vi "Get Status.vi"(8 "error in (no error)":errorcluster, 10 "Header Contents in":T1={"FILENAME"=["FILENAME", "example.fits", "File name at acquisition"], "OBSERVER"=["OBSERVER", "ECHARPE", "PI name"], "PROGRID"=["PROGRID", "UNDEFINED", "Program ID"], "OBJECT"=["OBJECT", "UNDEFINED", "Object name"], "NIGHTDIR"=["NIGHTDIR", "C:\\Users\\Sparc4_2\\Desktop\\Software Echarpe\\Imagens", "Night directory name "], "CHANNEL"=["CHANNEL", "RED", "Instrument channel"], "INSTRUME"=["INSTRUME", "ECHARPE", "Instrument"], "NEXPSEQ"=["NEXPSEQ", "1", "Total number of exposures in sequence"], "SEQINDEX"=["SEQINDEX", "1", "Exposure index in the sequence"], "OBSTYPE"=["OBSTYPE", "BIAS", "Image type: OBJECT, BIAS, FLAT, ARC, DARK"], "READMOD"=["READMOD", "Normal", "Read out mode: fast, normal, slow"], "SHUTTER"=["SHUTTER", "CLOSED", "Shutter Mode (OPEN, CLOSED, or AUTO) "], "OPENSHT"=["OPENSHT", "50", "Time to open the shutter (ms) "], "CLOSESHT"=["CLOSESHT", "50", "Time to close the shutter (ms)"], "GAIN"=["GAIN", "3.38", "Gain (e-/ADU)"], "GAINERR "=["GAINERR", "0.05", " Gain error (e-/ADU)"], "RDNOISE"=["RDNOISE", "6.55", "Read noise (e-)"], "RNOISERR"=["RNOISERR", "0.02", "Read noise error (e-)"], "SKYFIBER"=["SKYFIBER", "OFF", "Sky fiber: ON or OFF"], "CALFIBER"=["CALFIBER", "OFF", "Calibration Fiber: ON or OFF"], "UTDATE"=["UTDATE", "2017-10-01T20", "UT date at start of exposure"], "LOCTIME"=["LOCTIME", "2017-10-01T17", "LT date at start of exposure"], "MJD"=["MJD", "58027.500000", "Modified Julian Date at start of exposure"], "OBSLON"=["OBSLON", "-45.57972", "Observatory East Longitude"], "OBSLAT"=["OBSLAT", "-22.53444", "Observatory Latitude"], "OBSALT"=["OBSALT", "1864.0", "Observatory elevation above sea level (m)"], "EXPTIME"=["EXPTIME", "1", "Exposure time (s)"], "TELRA"=["TELRA", "", "TCS right ascension: HH:MM:SS.SSS"], "TELDEC"=["TELDEC", "", "TCS declination: “+-DD:MM:SS.SSS”"], "RA"=["RA", "00:00:00.000", "Requested right Ascension: HH:MM:SS.SSS"], "DEC"=["DEC", "+00:00:00.000", "Requested Declination: +- DD:MM:SS.SSS"], "RA_DEG"=["RA_DEG", "", "Requested Right Ascension (deg)"], "DEC_DEG"=["DEC_DEG", "", "Requested Declination (deg)"], "EPOCH"=["EPOCH", "", "Epoch for Target coordinates"], "HA"=["HA", "+01:13:05.98", "Hour Angle (Sexagesimal)"], "HAD"=["HAD", "", "Hour Angle (deg)"], "AIRMASS"=["AIRMASS", "1.085", "Mean airmass for the observation"], "AMSTART"=["AMSTART", "", "Airmass at start of exposure"], "AMEND"=["AMEND", "", "Airmass at end of exposure"], "XOFFSET"=["XOFFSET", "", "Telescope RA offset in arcsec"], "YOFFSET"=["YOFFSET", "", "Telescope DEC offset in arcsec"], "PA"=["PA", "14.6415392418", "Current Rotator Position Angle (degree)"], "CAMFOC"=["CAMFOC", "-3.53", "Camera focus position (mm)"], "TELFOC"=["TELFOC", "-3.53", "Telescope focus position (mm)"], "TCSUT"=["TCSUT", "", "TCS Universal Time"], "MOONDIST"=["MOONDIST", "", "Moon angular distance to object (deg)"], "MOONALT"=["MOONALT", "", "Moon elevation above horizon (deg)"], "MONNPHAS"=["MOONPHAS", "2017-10-01T20:34:3 6.000", "Moon phase (deg)"], "ADC"=["ADC", "ON", "Atmospheric Dispersion Corrector: ON or OFF"], "ADCSPPED"=["ADCSPPED", "5.0", "ADC motor speed (rpm)"], "CALMIRR"=["CALMIRR", "OUT", "Calibration mirror position: IN or OUT"], "GUIDING"=["GUIDING", "ON", "Guider status: ON or OFF"], "GUIDTEXP"=["GUIDTEXP", "1.0", "Guider exposure time (s)"], "GUIDFREQ"=["GUIDFREQ", "1.0", "Guiding frequency (Hz)"], "GUIDOBJX"=["GUIDOBJX", "102.5", "Guiding object x position (pixel)"], "GUIDOBJY"=["GUIDOBJY", "300.3", "Guiding object y position (pixel)"], "AVGYCORR"=["AVGYCORR", "2.3", "Average correction in RA (arcsec)"], "AVGXCORR"=["AVGXCORR", "1.3", "Average correction in DEC (arcsec)"], "GFOCUS"=["GFOCUS", "3.0", "Guider focus position (mm)"], "THARLAMP"=["THARLAMP", "OFF", "Thorium-Argon lamp state: ON or OFF"], "HALLAMP"=["HALLAMP", "OFF", "Halogen lamp state: ON or OFF"], "AGITATOR"=["AGITATOR", "ON", "Fiber agitator: ON or OFF"], "THARMIRR"=["THARMIRR", "SPECTROGRAPH", "Th-Ar mirror position: SPECTROGRAPH or TELESCOPE"], "DSTATUS"=["DSTATUS", "OPEN", "Dome Status: OPEN or CLOSED"], "DTEMP"=["DTEMP", "10.0", "Dome temperature (deg C)"], "DHUM"=["DHUM", "82.0", "Dome humidity (per cent)"], "DLAMP"=["DLAMP", "OFF", "Dome lamp: ON or OFF"], "DFLAT"=["DFLAT", "OFF", "Dome flat lamp: ON or OFF"], "TEMPEXT"=["TEMPEXT", "10.0", "External temperature (deg C)"], "PRESSURE"=["PRESSURE", "742.00", "Pressure (mbar)"], "HUMIDITY"=["HUMIDITY", "92.00", "Humidity (per cent)"], "WINDDIR"=["WINDDIR", "15.0", "Wind direction: North-eastward (deg)"], "WSPEED"=["WSPEED", "30.2", "Wind Speed (km/h)"], "TCSST"=["TCSST", "2017-10-01T20:34:3 6.000", "TCS Sideral Time"], "DPOS"=["DPOS", "0.00000", "Dome position (deg)"]}, 11 "TCS in":refnum<class "TCS.lvclass">) -> (0 "error out":errorcluster, 2 "Header Contents out":T1={"FILENAME"=["FILENAME", "example.fits", "File name at acquisition"], "OBSERVER"=["OBSERVER", "ECHARPE", "PI name"], "PROGRID"=["PROGRID", "UNDEFINED", "Program ID"], "OBJECT"=["OBJECT", "UNDEFINED", "Object name"], "NIGHTDIR"=["NIGHTDIR", "C:\\Users\\Sparc4_2\\Desktop\\Software Echarpe\\Imagens", "Night directory name "], "CHANNEL"=["CHANNEL", "RED", "Instrument channel"], "INSTRUME"=["INSTRUME", "ECHARPE", "Instrument"], "NEXPSEQ"=["NEXPSEQ", "1", "Total number of exposures in sequence"], "SEQINDEX"=["SEQINDEX", "1", "Exposure index in the sequence"], "OBSTYPE"=["OBSTYPE", "BIAS", "Image type: OBJECT, BIAS, FLAT, ARC, DARK"], "READMOD"=["READMOD", "Normal", "Read out mode: fast, normal, slow"], "SHUTTER"=["SHUTTER", "CLOSED", "Shutter Mode (OPEN, CLOSED, or AUTO) "], "OPENSHT"=["OPENSHT", "50", "Time to open the shutter (ms) "], "CLOSESHT"=["CLOSESHT", "50", "Time to close the shutter (ms)"], "GAIN"=["GAIN", "3.38", "Gain (e-/ADU)"], "GAINERR "=["GAINERR", "0.05", " Gain error (e-/ADU)"], "RDNOISE"=["RDNOISE", "6.55", "Read noise (e-)"], "RNOISERR"=["RNOISERR", "0.02", "Read noise error (e-)"], "SKYFIBER"=["SKYFIBER", "OFF", "Sky fiber: ON or OFF"], "CALFIBER"=["CALFIBER", "OFF", "Calibration Fiber: ON or OFF"], "UTDATE"=["UTDATE", "2017-10-01T20", "UT date at start of exposure"], "LOCTIME"=["LOCTIME", "2017-10-01T17", "LT date at start of exposure"], "MJD"=["MJD", "58027.500000", "Modified Julian Date at start of exposure"], "OBSLON"=["OBSLON", "-45.57972", "Observatory East Longitude"], "OBSLAT"=["OBSLAT", "-22.53444", "Observatory Latitude"], "OBSALT"=["OBSALT", "1864.0", "Observatory elevation above sea level (m)"], "EXPTIME"=["EXPTIME", "1", "Exposure time (s)"], "TELRA"=["TELRA", "", "TCS right ascension: HH:MM:SS.SSS"], "TELDEC"=["TELDEC", "", "TCS declination: “+-DD:MM:SS.SSS”"], "RA"=["RA", "00:00:00.000", "Requested right Ascension: HH:MM:SS.SSS"], "DEC"=["DEC", "+00:00:00.000", "Requested Declination: +- DD:MM:SS.SSS"], "RA_DEG"=["RA_DEG", "", "Requested Right Ascension (deg)"], "DEC_DEG"=["DEC_DEG", "", "Requested Declination (deg)"], "EPOCH"=["EPOCH", "", "Epoch for Target coordinates"], "HA"=["HA", "+01:13:05.98", "Hour Angle (Sexagesimal)"], "HAD"=["HAD", "", "Hour Angle (deg)"], "AIRMASS"=["AIRMASS", "1.085", "Mean airmass for the observation"], "AMSTART"=["AMSTART", "", "Airmass at start of exposure"], "AMEND"=["AMEND", "", "Airmass at end of exposure"], "XOFFSET"=["XOFFSET", "", "Telescope RA offset in arcsec"], "YOFFSET"=["YOFFSET", "", "Telescope DEC offset in arcsec"], "PA"=["PA", "14.6415392418", "Current Rotator Position Angle (degree)"], "CAMFOC"=["CAMFOC", "-3.53", "Camera focus position (mm)"], "TELFOC"=["TELFOC", "-3.53", "Telescope focus position (mm)"], "TCSUT"=["TCSUT", "", "TCS Universal Time"], "MOONDIST"=["MOONDIST", "", "Moon angular distance to object (deg)"], "MOONALT"=["MOONALT", "", "Moon elevation above horizon (deg)"], "MONNPHAS"=["MOONPHAS", "2017-10-01T20:34:3 6.000", "Moon phase (deg)"], "ADC"=["ADC", "ON", "Atmospheric Dispersion Corrector: ON or OFF"], "ADCSPPED"=["ADCSPPED", "5.0", "ADC motor speed (rpm)"], "CALMIRR"=["CALMIRR", "OUT", "Calibration mirror position: IN or OUT"], "GUIDING"=["GUIDING", "ON", "Guider status: ON or OFF"], "GUIDTEXP"=["GUIDTEXP", "1.0", "Guider exposure time (s)"], "GUIDFREQ"=["GUIDFREQ", "1.0", "Guiding frequency (Hz)"], "GUIDOBJX"=["GUIDOBJX", "102.5", "Guiding object x position (pixel)"], "GUIDOBJY"=["GUIDOBJY", "300.3", "Guiding object y position (pixel)"], "AVGYCORR"=["AVGYCORR", "2.3", "Average correction in RA (arcsec)"], "AVGXCORR"=["AVGXCORR", "1.3", "Average correction in DEC (arcsec)"], "GFOCUS"=["GFOCUS", "3.0", "Guider focus position (mm)"], "THARLAMP"=["THARLAMP", "OFF", "Thorium-Argon lamp state: ON or OFF"], "HALLAMP"=["HALLAMP", "OFF", "Halogen lamp state: ON or OFF"], "AGITATOR"=["AGITATOR", "ON", "Fiber agitator: ON or OFF"], "THARMIRR"=["THARMIRR", "SPECTROGRAPH", "Th-Ar mirror position: SPECTROGRAPH or TELESCOPE"], "DSTATUS"=["DSTATUS", "OPEN", "Dome Status: OPEN or CLOSED"], "DTEMP"=["DTEMP", "10.0", "Dome temperature (deg C)"], "DHUM"=["DHUM", "82.0", "Dome humidity (per cent)"], "DLAMP"=["DLAMP", "OFF", "Dome lamp: ON or OFF"], "DFLAT"=["DFLAT", "OFF", "Dome flat lamp: ON or OFF"], "TEMPEXT"=["TEMPEXT", "10.0", "External temperature (deg C)"], "PRESSURE"=["PRESSURE", "742.00", "Pressure (mbar)"], "HUMIDITY"=["HUMIDITY", "92.00", "Humidity (per cent)"], "WINDDIR"=["WINDDIR", "15.0", "Wind direction: North-eastward (deg)"], "WSPEED"=["WSPEED", "30.2", "Wind Speed (km/h)"], "TCSST"=["TCSST", "2017-10-01T20:34:3 6.000", "TCS Sideral Time"], "DPOS"=["DPOS", "0.00000", "Dome position (deg)"]}, 3 "TCS out":refnum<class "TCS.lvclass">)   [LabVIEW 2018, in "TCS.lvclass"]
uses:
  TCS.lvclass
  TCS.lvclass/TCS.ctl
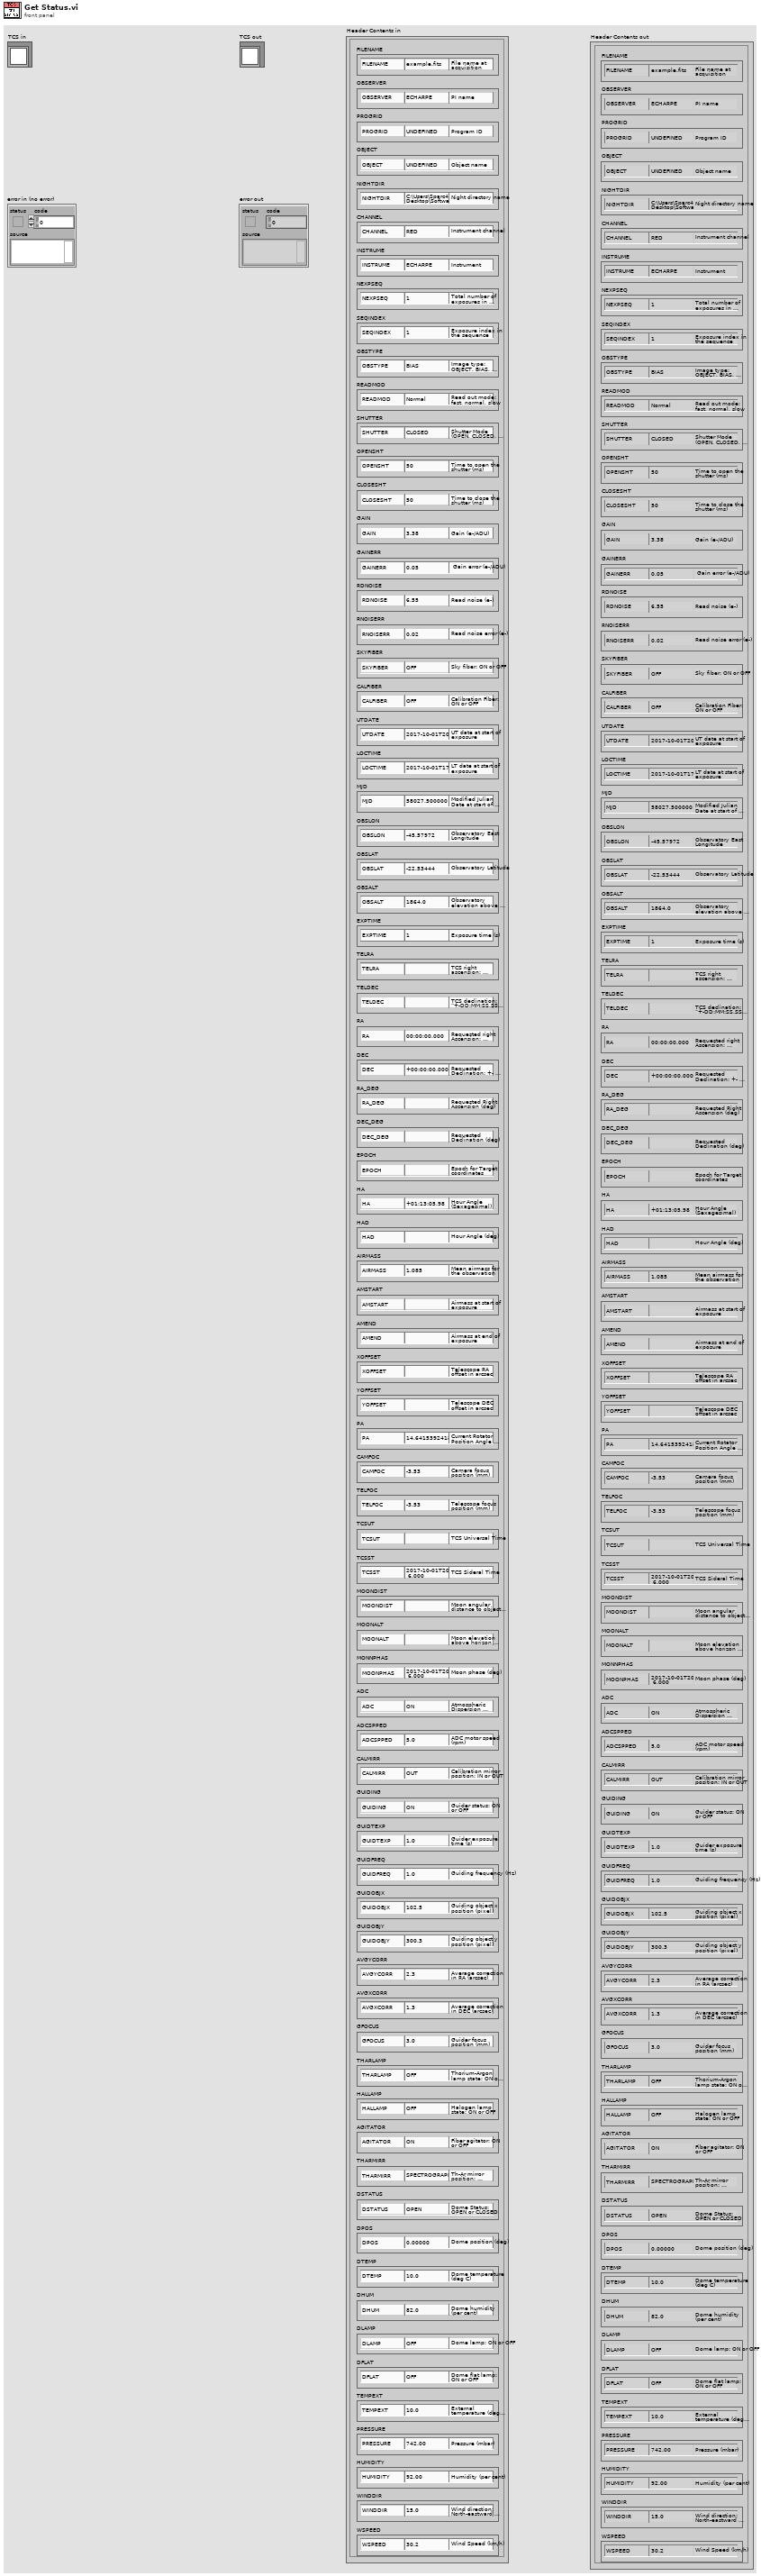
[diagram p1: front panel]
types:
  T1 = cluster{"FILENAME":string[], "OBSERVER":string[], "PROGRID":string[], "OBJECT":string[], "NIGHTDIR":string[], "CHANNEL":string[], "INSTRUME":string[], "NEXPSEQ":string[], "SEQINDEX":string[], "OBSTYPE":string[], "READMOD":string[], "SHUTTER":string[], "OPENSHT":string[], "CLOSESHT":string[], "GAIN":string[], "GAINERR ":string[], "RDNOISE":string[], "RNOISERR":string[], "SKYFIBER":string[], "CALFIBER":string[], "UTDATE":string[], "LOCTIME":string[], "MJD":string[], "OBSLON":string[], "OBSLAT":string[], "OBSALT":string[], "EXPTIME":string[], "TELRA":string[], "TELDEC":string[], "RA":string[], "DEC":string[], "RA_DEG":string[], "DEC_DEG":string[], "EPOCH":string[], "HA":string[], "HAD":string[], "AIRMASS":string[], "AMSTART":string[], "AMEND":string[], "XOFFSET":string[], "YOFFSET":string[], "PA":string[], "CAMFOC":string[], "TELFOC":string[], "TCSUT":string[], "MOONDIST":string[], "MOONALT":string[], "MONNPHAS":string[], "ADC":string[], "ADCSPPED":string[], "CALMIRR":string[], "GUIDING":string[], "GUIDTEXP":string[], "GUIDFREQ":string[], "GUIDOBJX":string[], "GUIDOBJY":string[], "AVGYCORR":string[], "AVGXCORR":string[], "GFOCUS":string[], "THARLAMP":string[], "HALLAMP":string[], "AGITATOR":string[], "THARMIRR":string[], "DSTATUS":string[], "DTEMP":string[], "DHUM":string[], "DLAMP":string[], "DFLAT":string[], "TEMPEXT":string[], "PRESSURE":string[], "HUMIDITY":string[], "WINDDIR":string[], "WSPEED":string[], "TCSST":string[], "DPOS":string[]}
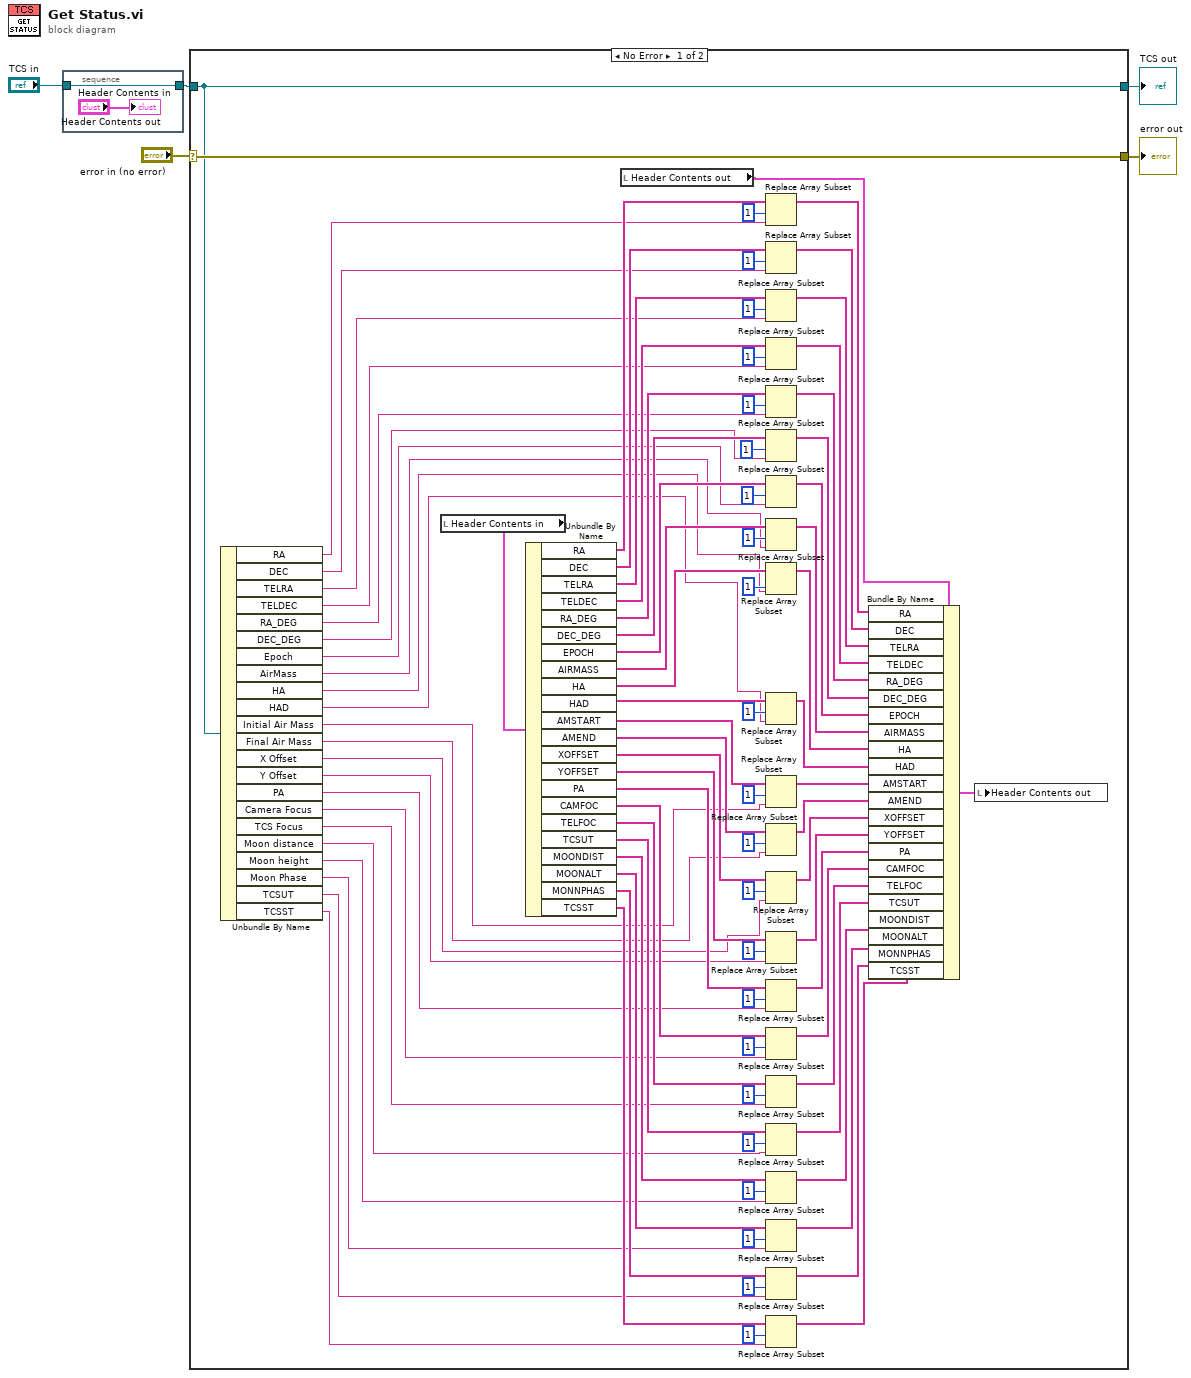
[diagram p0: block diagram]
diagram:
  n1 = stacked-sequence {
    tunnel: "TCS in" -> [w7]
    tunnel: [w7] -> w2
    frame #0 {
      "Header Contents out" <- "Header Contents in"
    }
  }
  n2 = case shown="No Error" "error in (no error)" {
    selector: "error in (no error)" -> [w100 w102]
    tunnel: [w100 w102] -> w5
    tunnel: [w99 w101] -> w4
    tunnel: w2 -> [w99 w101]
    frame No Error {
      n3 = Unbundle By Name(w99) -> ("RA"=w32:string, "DEC"=w31:string, "TELRA"=w30:string, "TELDEC"=w29:string, "RA_DEG"=w28:string, "DEC_DEG"=w27:string, "Epoch"=w26:string, "AirMass"=w25:string, "HA"=w24:string, "HAD"=w23:string, "Initial Air Mass"=w11:string, "Final Air Mass"=w12:string, "X Offset"=w13:string, "Y Offset"=w14:string, "PA"=w15:string, "Camera Focus"=w16:string, "TCS Focus"=w17:string, "Moon distance"=w18:string, "Moon height"=w19:string, "Moon Phase"=w20:string, "TCSUT"=w21:string, "TCSST"=w22:string)
      n4 = local read "Header Contents in"() -> (w9:T1)
      n5 = Unbundle By Name(w9) -> ("RA"=w67:string[], "DEC"=w66:string[], "TELRA"=w65:string[], "TELDEC"=w64:string[], "RA_DEG"=w63:string[], "DEC_DEG"=w62:string[], "EPOCH"=w61:string[], "AIRMASS"=w60:string[], "HA"=w59:string[], "HAD"=w58:string[], "AMSTART"=w57:string[], "AMEND"=w56:string[], "XOFFSET"=w55:string[], "YOFFSET"=w54:string[], "PA"=w53:string[], "CAMFOC"=w52:string[], "TELFOC"=w46:string[], "TCSUT"=w43:string[], "MOONDIST"=w42:string[], "MOONALT"=w41:string[], "MONNPHAS"=w40:string[], "TCSST"=w38:string[])
      n6 = local read "Header Contents out"() -> (w10:T1)
      n7 = Replace Array Subset(array=w67, new element=w32, index=1) -> (w82:string[])
      n8 = Replace Array Subset(array=w66, new element=w31, index=1) -> (w81:string[])
      n9 = Replace Array Subset(array=w65, new element=w30, index=1) -> (w80:string[])
      n10 = Replace Array Subset(array=w64, new element=w29, index=1) -> (w79:string[])
      n11 = Replace Array Subset(array=w63, new element=w28, index=1) -> (w78:string[])
      n12 = Replace Array Subset(array=w62, new element=w27, index=1) -> (w77:string[])
      n13 = Replace Array Subset(array=w61, new element=w26, index=1) -> (w76:string[])
      n14 = Replace Array Subset(array=w60, new element=w25, index=1) -> (w75:string[])
      n15 = Replace Array Subset(array=w59, new element=w24, index=1) -> (w74:string[])
      n16 = Replace Array Subset(array=w58, new element=w23, index=1) -> (w73:string[])
      n17 = Replace Array Subset(array=w57, new element=w11, index=1) -> (w72:string[])
      n18 = Replace Array Subset(array=w56, new element=w12, index=1) -> (w71:string[])
      n19 = Replace Array Subset(array=w55, new element=w13, index=1) -> (w70:string[])
      n20 = Replace Array Subset(array=w54, new element=w14, index=1) -> (w69:string[])
      n21 = Replace Array Subset(array=w53, new element=w15, index=1) -> (w68:string[])
      n22 = Replace Array Subset(array=w52, new element=w16, index=1) -> (w45:string[])
      n23 = Replace Array Subset(array=w46, new element=w17, index=1) -> (w44:string[])
      n24 = Replace Array Subset(array=w43, new element=w18, index=1) -> (w37:string[])
      n25 = Replace Array Subset(array=w42, new element=w19, index=1) -> (w36:string[])
      n26 = Replace Array Subset(array=w41, new element=w20, index=1) -> (w35:string[])
      n27 = Replace Array Subset(array=w40, new element=w21, index=1) -> (w34:string[])
      n28 = Replace Array Subset(array=w38, new element=w22, index=1) -> (w33:string[])
      n29 = Bundle By Name(cluster=w10, "RA"=w82, "DEC"=w81, "TELRA"=w80, "TELDEC"=w79, "RA_DEG"=w78, "DEC_DEG"=w77, "EPOCH"=w76, "AIRMASS"=w75, "HA"=w74, "HAD"=w73, "AMSTART"=w72, "AMEND"=w71, "XOFFSET"=w70, "YOFFSET"=w69, "PA"=w68, "CAMFOC"=w45, "TELFOC"=w44, "TCSUT"=w37, "MOONDIST"=w36, "MOONALT"=w35, "MONNPHAS"=w34, "TCSST"=w33) -> (w8:T1)
      n30 = local write "Header Contents out"(w8) -> ()
    }
    frame Error {
    }
  }
  "error out" <- w5
  "TCS out" <- w4
